vi "Build Test Sequence.vi"(8 "error in":errorcluster, 11 "Configured Steps In":T1[](array[typedef])) -> (0 "error out":errorcluster, 3 "Configured Steps Out":T1[](array[typedef]))   [LabVIEW 2018]
doc: "This VI provides a UI to build, configure, and modify a real-time control sequence."
uses:
  controls/Configured Step.ctl
  controls/VI Reference Type.ctl
panel:
  in  "Save":bool
  in  "Load":bool
  in  "Cancel Button":bool
  in  "Move Down":bool
  in  "Move Up":bool
  in  "Done":bool
  in  "Add Step":bool
  in  "Remove Step":bool
  in  "Control Sequence":i32(listbox)
  in  "Available Steps":i32(listbox)
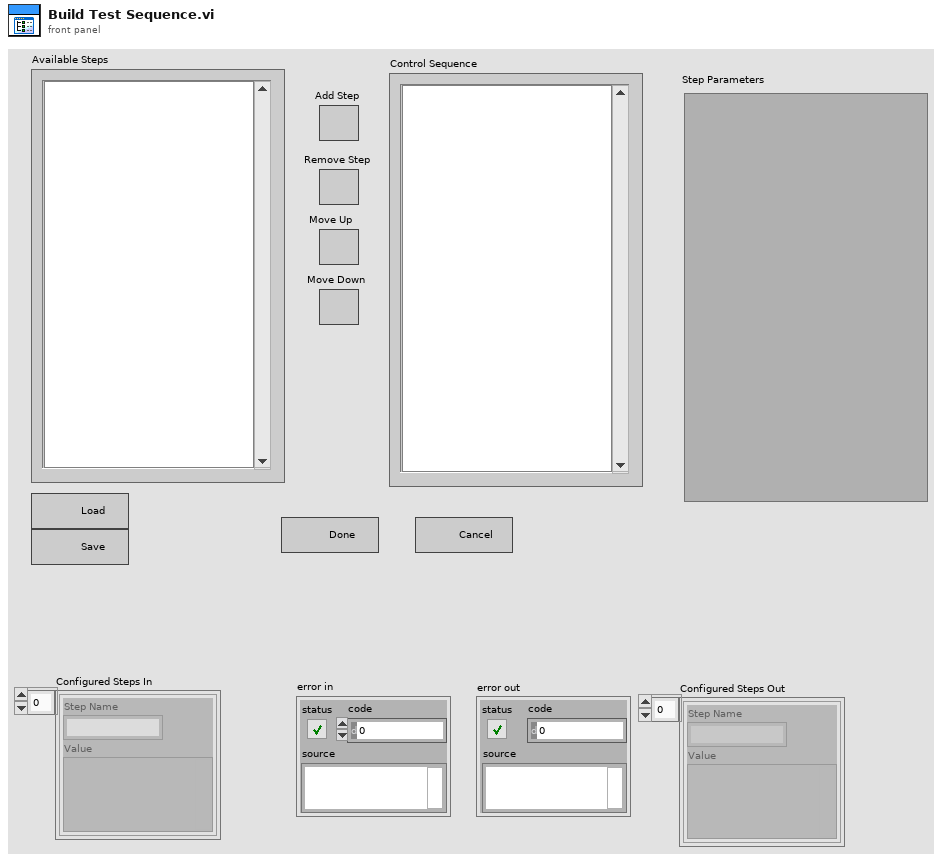
[diagram p1: front panel]
types:
  T1 = typedef "Configured Step.ctl" = cluster{"Step Name":string, "Value":variant}
  T2 = typedef "VI Reference Type.ctl" = refnum<vi>
  T3 = enum16{"open", "replace", "create", "open or create", "replace or create", "replace or create with confirmation"}
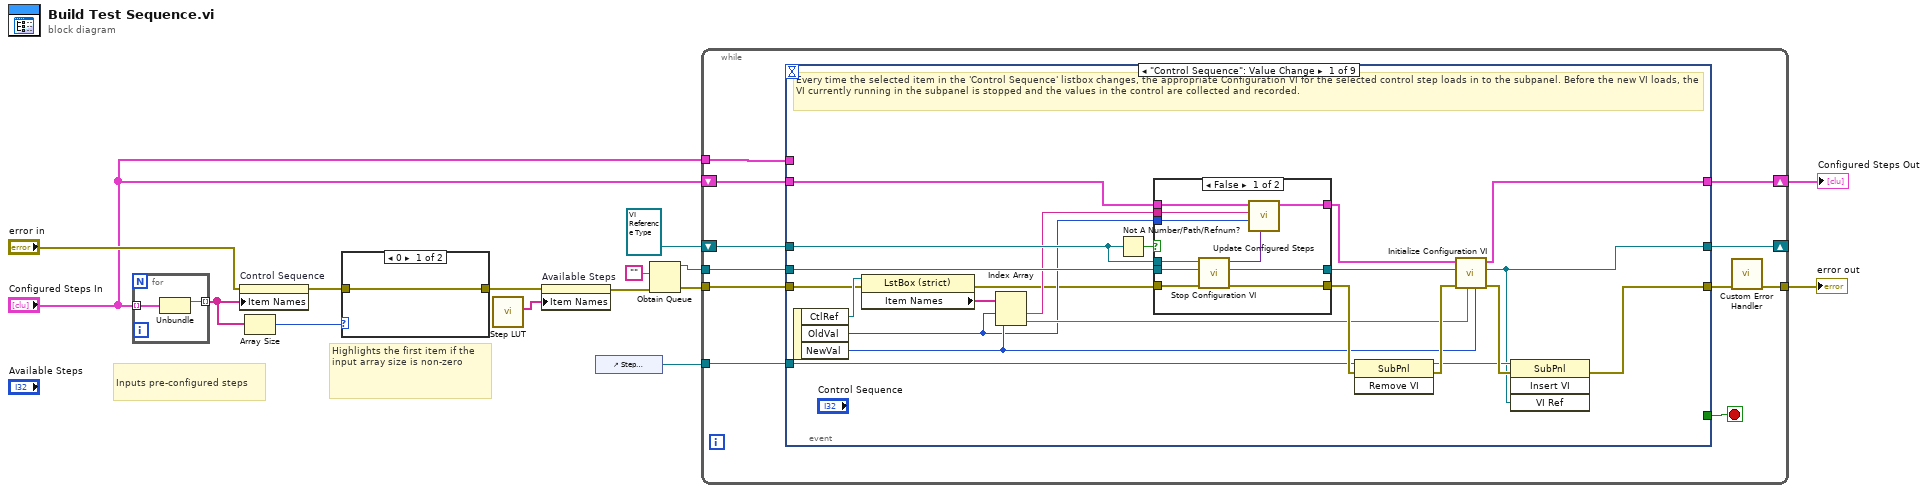
[diagram p0: block diagram]
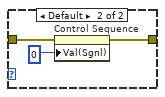
[diagram p2: hidden frame]
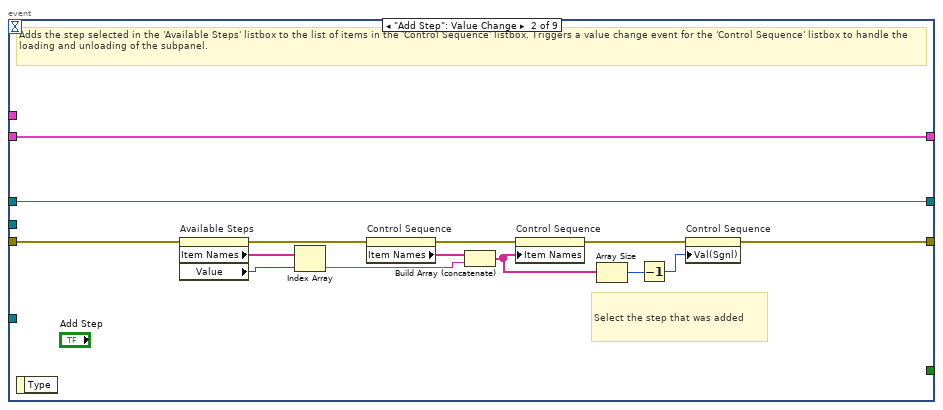
[diagram p4: hidden frame]
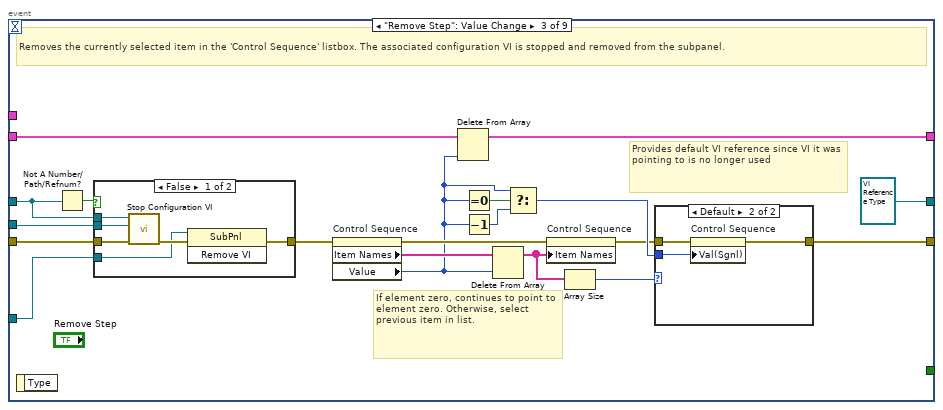
[diagram p5: hidden frame]
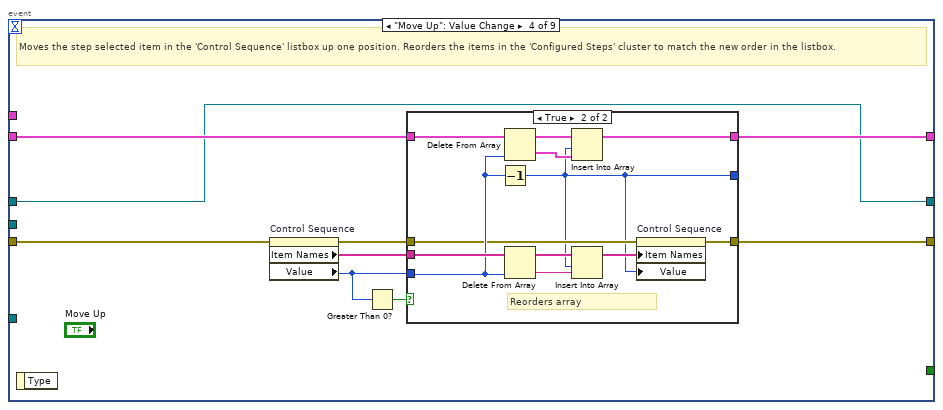
[diagram p8: hidden frame]
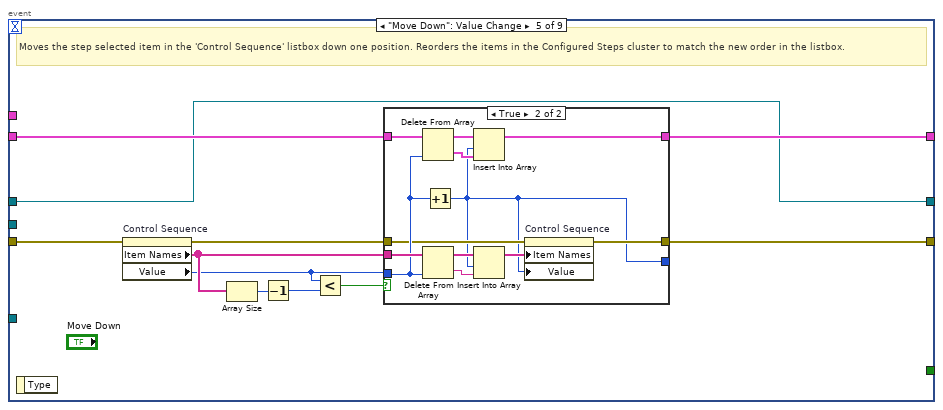
[diagram p10: hidden frame]
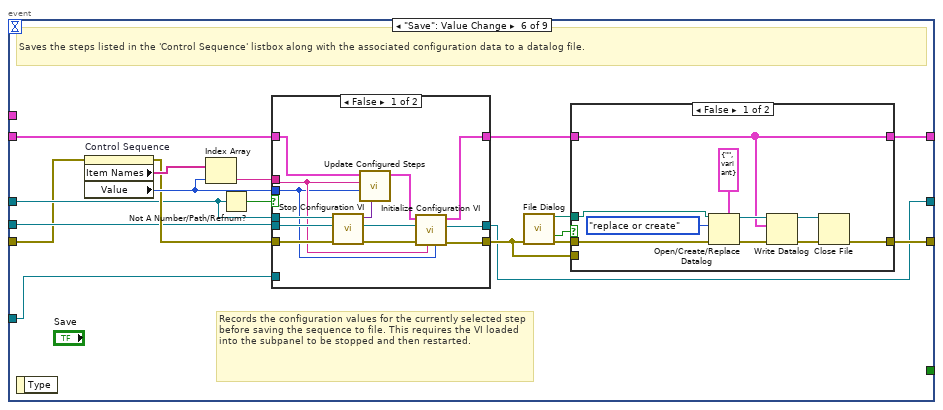
[diagram p12: hidden frame]
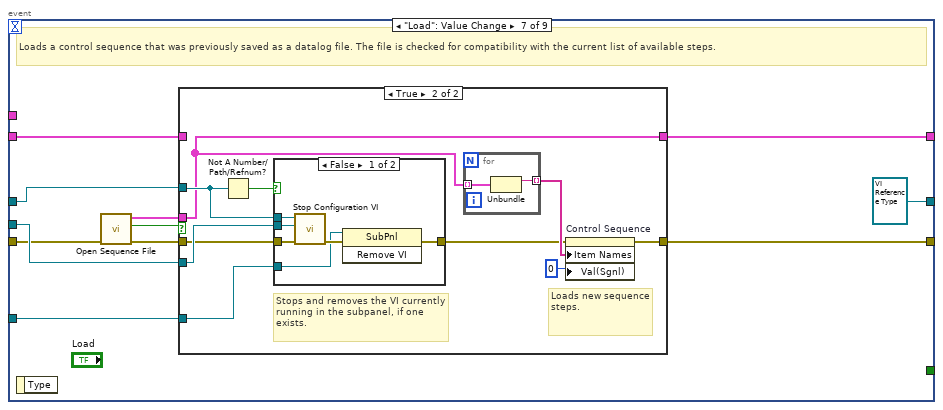
[diagram p15: hidden frame]
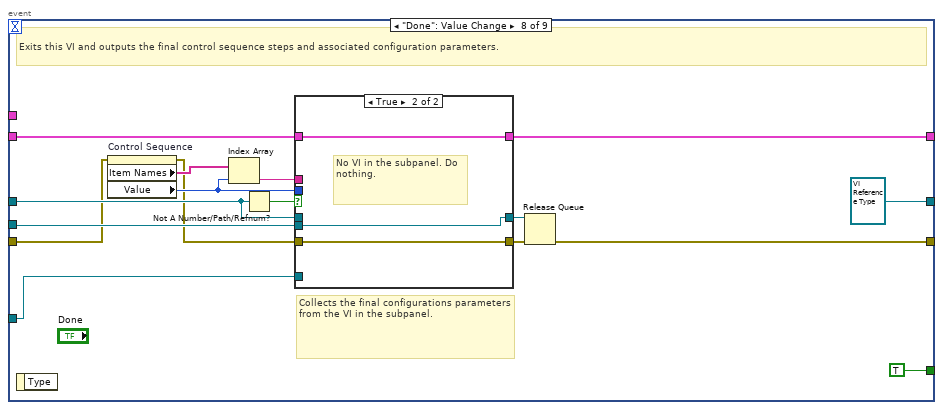
[diagram p18: hidden frame]
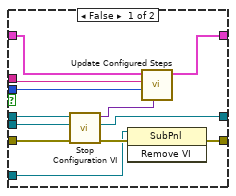
[diagram p19: hidden frame]
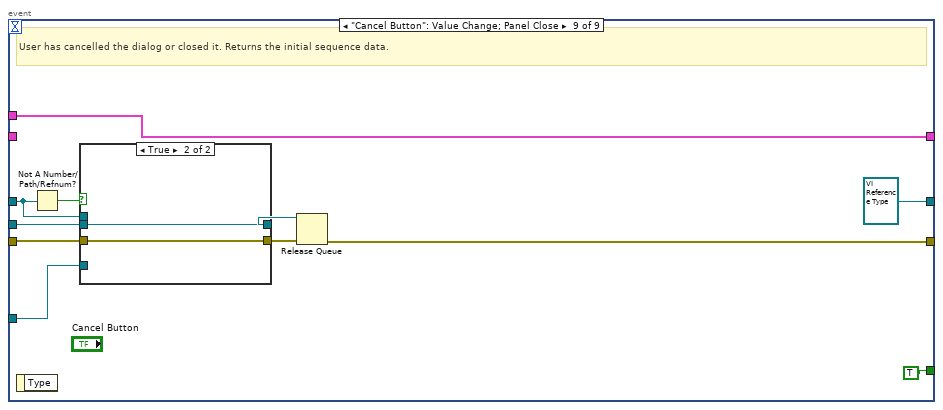
[diagram p20: hidden frame]
diagram:
  # "Highlights the first item if the input array size is non-zero"
  # "Inputs pre-configured steps"
  n1 = for {
    tunnel: "Configured Steps In" -> [w17] mode=indexing
    tunnel: [w16] -> w13 mode=indexing
    n2 = Unbundle(w17) -> ("Step Name"=w16:string)  [unwired: 1 out]
  }
  n3 = property on="Control Sequence" class="LstBox (strict)"(error in="error in", "Item Names"=w13) -> (error out=w10:errorcluster)  [unwired: 1 in, 1 out]
  n4 = Array Size(array=w13) -> (size(s)=w1:i32)
  n5 = case shown="0" w1 {
    tunnel: w10 -> [w18 w20]
    tunnel: [w18 w19] -> w9
    frame 0 {
    }
    frame Default {
      n6 = property on="Control Sequence" class="LstBox (strict)"(error in=w20, "Val(Sgnl)"=0 ("Value (Signaling)")) -> (error out=w19:errorcluster)  [unwired: 1 in, 1 out]
    }
  }
  n7 = call "Step LUT.vi"() -> ("Available Steps"=w8:string[])  [unwired: 10 in, 1 out]
  n8 = property on="Available Steps" class="LstBox (strict)"(error in=w9, "Item Names"=w8) -> (error out=w7:errorcluster)  [unwired: 1 in, 1 out]
  n9 = control-ref of="Step Parameters"() -> (w14:refnum<vi>)
  n10 = Obtain Queue(element data type="", error in (no error)=w7) -> (queue out=w4:refnum<queue>, error out=w6:errorcluster)  [unwired: 3 in, 1 out]
  n11 = while {
    shift-right: [w25] -> _
    shift-left: T2 refnum ("VI reference") -> [w31]
    shift-right: [w30] -> w12
    shift-left: "Configured Steps In" -> [w29]
    tunnel: w14 -> [w22]
    tunnel: "Configured Steps In" -> [w27]
    tunnel: w4 -> [w26]
    tunnel: w6 -> [w28]
    tunnel: [w23] -> w15
    stop <- w32 stop-if-true
    n12 = event shown="[0] \"Control Sequence\": Value Change" {
      selector: _ -> [_ _ _ _ _ _ _ _ _]
      dyn-events: _ -> [_ _ _ _ _ _ _ _ _]
      timeout: _ -> [_ _ _ _ _ _ _ _ _]
      tunnel: [_ _ _ _ _ _ _ TRUE TRUE] -> w32
      tunnel: w31 -> [w51 w70 w91 w112 w139 w165 w213 w250 w276]
      tunnel: [w41 w79 w98 w117 w144 w175 w218 w248 w281] -> w30
      tunnel: w29 -> [w50 w79 w97 w118 w145 w168 w212 w247 _]
      tunnel: w28 -> [w39 w71 w89 w120 w146 w164 w211 w241 w275]
      tunnel: [w44 w75 w82 w115 w142 w179 w217 w254 w279] -> w24
      tunnel: w22 -> [w48 _ w88 _ _ w169 w216 w245 w274]
      tunnel: w27 -> [_ _ _ _ _ _ _ _ w281]
      tunnel: w26 -> [w43 _ w90 _ _ w166 w214 w251 w272]
      tunnel: [w40 w70 T2 refnum ("VI Reference out") w112 w139 w162 T2 refnum ("VI reference in") T2 refnum ("VI reference in") T2 refnum ("VI reference in")] -> w25
      event "Control Sequence": Value Change {
        # "Every time the selected item in the 'Control Sequence' listbox changes, the appropriate Configuration VI for the selected control step loads in to the subpanel. Before the new VI loads, the VI currently running in the subpanel is stopped and the values in the control are collected and recorded."
        n13 = event-data() -> ("CtlRef"=w54:refnum<vi>, "OldVal"=w35:i32, "NewVal"=w37:i32)  [unwired: 1 in]
        n14 = property class="LstBox (strict)"(reference=w54, error in=w39) -> (error out=w33:errorcluster, "Item Names"=w53:string[])  [unwired: 1 out]
        n15 = Index Array(array=w53, index #1=w35, index #2=w37) -> (element #1=w36:string, element #2=w38:string)
        n16 = Not A Number/Path/Refnum?(number/path/refnum=w51) -> (NaN/Path/Refnum?=w52:bool)
        n17 = case shown="False" w52 {
          tunnel: w51 -> [w64 _]
          tunnel: w36 -> [w59 _]
          tunnel: w50 -> [w56 w65]
          tunnel: [w62 w67] -> w49
          tunnel: w35 -> [w60 _]
          tunnel: w33 -> [w63 w67]
          tunnel: w43 -> [w61 w66]
          tunnel: [w58 w66] -> w42
          tunnel: [w55 w65] -> w34
          frame False {
            n18 = call "Stop Configuration VI.vi"("error in (no error)"=w63, "Subpanel Queue In"=w61, "VI in"=w64) -> ("error out"=w62:errorcluster, "Subpanel Queue Out"=w58:refnum<queue>, "Variant Out"=w57:variant)  [unwired: 6 in]
            n19 = call "Update Configured Steps.vi"("Parameters In"=w57, "Step Number"=w60, "Step Name"=w59, "Configured Steps In"=w56) -> ("Configured Steps Out"=w55:T1[])  [unwired: 7 in]
          }
          frame True {
            # "No VI currently loaded in the subpanel. Do nothing"
          }
        }
        n20 = invoke class="SubPnl" method="Remove VI"(reference=w48, error in=w49) -> (reference out=w45:refnum<vi>, error out=w47:errorcluster)  [unwired: 1 in, 1 out]
        n21 = call "Initialize Configuration VI.vi"("Step Number"=w37, "Step Name"=w38, "error in (no error)"=w47, "Subpanel Queue in"=w42, "Configured Steps In"=w34) -> ("error out"=w46:errorcluster, "VI Reference out"=w40:T2, "Configured Steps Out"=w41:T1[])  [unwired: 4 in]
        n22 = invoke on="Invoke Node" class="SubPnl" method="Insert VI"(reference=w45, error in=w46, "VI Ref"=w40) -> (error out=w44:errorcluster)  [unwired: 1 in, 3 out]
      }
      event "Add Step": Value Change {
        # "Select the step that was added"
        # "Adds the step selected in the 'Available Steps' listbox to the list of items in the 'Control Sequence' listbox. Triggers a value change event for the 'Control Sequence' listbox to handle the loading and unloading of the subpanel."
        n23 = event-data() -> ()  [unwired: 1 in, 1 out]
        n24 = property on="Available Steps" class="LstBox (strict)"(error in=w71) -> (error out=w78:errorcluster, "Item Names"=w72:string[], "Value"=w69:i32)  [unwired: 1 in, 1 out]
        n25 = Index Array(array=w72, index=w69) -> (element=w73:string)
        n26 = property on="Control Sequence" class="LstBox (strict)"(error in=w78) -> (error out=w77:errorcluster, "Item Names"=w81:string[])  [unwired: 1 in, 1 out]
        n27 = Build Array (concatenate)(w81, w73) -> (w68:string[])
        n28 = property on="Control Sequence" class="LstBox (strict)"(error in=w77, "Item Names"=w68) -> (error out=w76:errorcluster)  [unwired: 1 in, 1 out]
        n29 = Array Size(array=w68) -> (size(s)=w80:i32)
        n30 = Decrement(x=w80) -> (x-1=w74:i32)
        n31 = property on="Control Sequence" class="LstBox (strict)"(error in=w76, "Val(Sgnl)"=w74) -> (error out=w75:errorcluster)  [unwired: 1 in, 1 out]
      }
      event "Remove Step": Value Change {
        # "If element zero, continues to point to element zero. Otherwise, select previous item in list."
        # "Provides default VI reference since VI it was pointing to is no longer used"
        # "Removes the currently selected item in the 'Control Sequence' listbox. The associated configuration VI is stopped and removed from the subpanel."
        n32 = event-data() -> ()  [unwired: 1 in, 1 out]
        n33 = Not A Number/Path/Refnum?(number/path/refnum=w91) -> (NaN/Path/Refnum?=w92:bool)
        n34 = case shown="False" w92 {
          tunnel: w89 -> [w107 w111]
          tunnel: [w110 w111] -> w87
          tunnel: w91 -> [w109 _]
          tunnel: w90 -> [w108 _]
          tunnel: w88 -> [w105 _]
          frame False {
            n35 = call "Stop Configuration VI.vi"("error in (no error)"=w107, "Subpanel Queue In"=w108, "VI in"=w109) -> ("error out"=w106:errorcluster)  [unwired: 6 in, 2 out]
            n36 = invoke class="SubPnl" method="Remove VI"(reference=w105, error in=w106) -> (error out=w110:errorcluster)  [unwired: 1 in, 2 out]
          }
          frame True {
          }
        }
        n37 = property on="Control Sequence" class="LstBox (strict)"(error in=w87) -> (error out=w99:errorcluster, "Item Names"=w100:string[], "Value"=w95:i32)  [unwired: 1 in, 1 out]
        n38 = Delete From Array(array=w97, index=w95) -> (array with subset deleted=w98:T1[])  [unwired: 1 in, 1 out]
        n39 = Equal To 0?(x=w95) -> (x = 0?=w96:bool)
        n40 = Decrement(x=w95) -> (x-1=w94:i32)
        n41 = Delete From Array(array=w100, index=w95) -> (array with subset deleted=w86:string[])  [unwired: 1 in, 1 out]
        n42 = Select(t=w95, s=w96, f=w94) -> (s? t:f=w84:i32)
        n43 = property on="Control Sequence" class="LstBox (strict)"(error in=w99, "Item Names"=w86) -> (error out=w83:errorcluster)  [unwired: 1 in, 1 out]
        n44 = Array Size(array=w86) -> (size(s)=w85:i32)
        n45 = case shown="Default" w85 {
          tunnel: w84 -> [_ w104]
          tunnel: w83 -> [w101 w103]
          tunnel: [w101 w102] -> w82
          frame 0 {
            # "No elements in Control Sequence listbox. Do nothing."
          }
          frame Default {
            n46 = property on="Control Sequence" class="LstBox (strict)"(error in=w103, "Val(Sgnl)"=w104) -> (error out=w102:errorcluster)  [unwired: 1 in, 1 out]
          }
        }
      }
      event "Move Up": Value Change {
        # "Moves the step selected item in the 'Control Sequence' listbox up one position. Reorders the items in the 'Configured Steps' cluster to match the new order in the listbox."
        n47 = event-data() -> ()  [unwired: 1 in, 1 out]
        n48 = property on="Control Sequence" class="LstBox (strict)"(error in=w120) -> (error out=w116:errorcluster, "Item Names"=w119:string[], "Value"=w113:i32)  [unwired: 1 in, 1 out]
        n49 = Greater Than 0?(x=w113) -> (x > 0?=w114:bool)
        n50 = case shown="True" w114 {
          tunnel: w119 -> [_ w135]
          tunnel: w118 -> [w121 w134]
          tunnel: w113 -> [w122 w131]
          tunnel: [w121 w128] -> w117
          tunnel: w116 -> [w123 w127]
          tunnel: [w123 w125] -> w115
          tunnel: [w122 w124] -> _
          frame False {
            # "Selected item is already at the top of the list. Do nothing."
          }
          frame True {
            # "Reorders array"
            n51 = Decrement(x=w131) -> (x-1=w124:i32)
            n52 = Delete From Array(array=w134, index=w131) -> (deleted portion=w129:T1, array with subset deleted=w130:T1[])  [unwired: 1 in]
            n53 = Delete From Array(array=w135, index=w131) -> (deleted portion=w132:string, array with subset deleted=w133:string[])  [unwired: 1 in]
            n54 = Insert Into Array(array=w130, index=w124, new element=w129) -> (w128:T1[])
            n55 = Insert Into Array(array=w133, index=w124, new element=w132) -> (w126:string[])
            n56 = property on="Control Sequence" class="LstBox (strict)"(error in=w127, "Item Names"=w126, "Value"=w124) -> (error out=w125:errorcluster)  [unwired: 1 in, 1 out]
          }
        }
      }
      event "Move Down": Value Change {
        # "Moves the step selected item in the 'Control Sequence' listbox down one position. Reorders the items in the Configured Steps cluster to match the new order in the listbox."
        n57 = event-data() -> ()  [unwired: 1 in, 1 out]
        n58 = property on="Control Sequence" class="LstBox (strict)"(error in=w146) -> (error out=w143:errorcluster, "Item Names"=w140:string[], "Value"=w138:i32)  [unwired: 1 in, 1 out]
        n59 = Array Size(array=w140) -> (size(s)=w141:i32)
        n60 = Decrement(x=w141) -> (x-1=w137:i32)
        n61 = Less?(x=w138, y=w137) -> (x < y?=w136:bool)
        n62 = case shown="True" w136 {
          tunnel: w140 -> [_ w161]
          tunnel: w145 -> [w147 w160]
          tunnel: w138 -> [w148 w157]
          tunnel: [w147 w154] -> w144
          tunnel: w143 -> [w149 w153]
          tunnel: [w149 w151] -> w142
          tunnel: [w148 w150] -> _
          frame False {
            # "Selected item is already the last item in the list. Do nothing."
          }
          frame True {
            n63 = Delete From Array(array=w160, index=w157) -> (deleted portion=w155:T1, array with subset deleted=w156:T1[])  [unwired: 1 in]
            n64 = Delete From Array(array=w161, index=w157) -> (deleted portion=w158:string, array with subset deleted=w159:string[])  [unwired: 1 in]
            n65 = Increment(x=w157) -> (x+1=w150:i32)
            n66 = Insert Into Array(array=w156, index=w150, new element=w155) -> (w154:T1[])
            n67 = Insert Into Array(array=w159, index=w150, new element=w158) -> (w152:string[])
            n68 = property on="Control Sequence" class="LstBox (strict)"(error in=w153, "Item Names"=w152, "Value"=w150) -> (error out=w151:errorcluster)  [unwired: 1 in, 1 out]
          }
        }
      }
      event "Save": Value Change {
        # "Records the configuration values for the currently selected step before saving the sequence to file. This requires the VI loaded into the subpanel to be stopped and then restarted."
        # "Saves the steps listed in the 'Control Sequence' listbox along with the associated configuration data to a datalog file."
        n69 = event-data() -> ()  [unwired: 1 in, 1 out]
        n70 = property on="Control Sequence" class="LstBox (strict)"(error in=w164) -> (error out=w170:errorcluster, "Item Names"=w173:string[], "Value"=w172:i32)  [unwired: 1 in, 1 out]
        n71 = Index Array(array=w173, index=w172) -> (element=w171:string)
        n72 = Not A Number/Path/Refnum?(number/path/refnum=w165) -> (NaN/Path/Refnum?=w174:bool)
        n73 = case shown="False" w174 {
          tunnel: w165 -> [w192 w193]
          tunnel: w171 -> [w184 _]
          tunnel: [w181 w195] -> w167
          tunnel: w168 -> [w188 w195]
          tunnel: [w182 w194] -> w163
          tunnel: w172 -> [w183 _]
          tunnel: w170 -> [w191 w194]
          tunnel: w166 -> [w190 _]
          tunnel: w169 -> [_ _]
          tunnel: [w180 w193] -> w162
          frame False {
            n74 = call "Stop Configuration VI.vi"("error in (no error)"=w191, "Subpanel Queue In"=w190, "VI in"=w192) -> ("error out"=w186:errorcluster, "Subpanel Queue Out"=w187:refnum<queue>, "Variant Out"=w189:variant)  [unwired: 6 in]
            n75 = call "Update Configured Steps.vi"("Parameters In"=w189, "Step Number"=w183, "Step Name"=w184, "Configured Steps In"=w188) -> ("Configured Steps Out"=w185:T1[])  [unwired: 7 in]
            n76 = call "Initialize Configuration VI.vi"("Step Number"=w183, "Step Name"=w184, "error in (no error)"=w186, "Subpanel Queue in"=w187, "Configured Steps In"=w185) -> ("error out"=w182:errorcluster, "VI Reference out"=w180:T2, "Configured Steps Out"=w181:T1[])  [unwired: 4 in]
          }
          frame True {
            # "Not a valid VI reference\n as an input. \nDo nothing"
          }
        }
        n77 = call "File Dialog"("error in"=w163) -> ("selected path"=w177:path, "cancelled"=w176:bool, "error out"=w178:errorcluster)  [unwired: 11 in, 1 out]
        n78 = case shown="False" w176 {
          tunnel: w167 -> [w196 w207]
          tunnel: [w199 w206] -> w179
          tunnel: w178 -> [w198 _]
          tunnel: w177 -> [w197 _]
          tunnel: [w196 w207] -> w175
          tunnel: w163 -> [_ w206]
          frame False {
            n79 = Open/Create/Replace Datalog(5:T1 {"Step Name"="", "Value"=variant} ("Configured Step"), 8:w198, 10:T3."replace or create" ("operation (0:open)"), 11:w197) -> (0:w205:errorcluster, 3:w202:refnum<k1>)  [unwired: 2 in, 1 out]
            n80 = Write Datalog(4:w205, 6:w196, 7:w202) -> (0:w201:errorcluster, 3:w200:refnum<k1>)
            n81 = Close File(refnum=w200, error in=w201) -> (error out=w199:errorcluster)  [unwired: 1 out]
          }
          frame True {
          }
        }
      }
      event "Load": Value Change {
        # "Loads a control sequence that was previously saved as a datalog file. The file is checked for compatibility with the current list of available steps."
        n82 = event-data() -> ()  [unwired: 1 in, 1 out]
        n83 = call "Open Sequence File.vi"("error in"=w211) -> ("error out"=w210:errorcluster, "Valid?"=w209:bool, "Configured Steps Out"=w208:T1[])  [unwired: 8 in]
        n84 = case shown="True" w209 {
          tunnel: [w220 w222] -> w218
          tunnel: [w219 w229] -> w217
          tunnel: w210 -> [w219 w221]
          tunnel: w212 -> [w220 _]
          tunnel: w216 -> [_ w223]
          tunnel: w214 -> [_ w228]
          tunnel: w213 -> [_ w227]
          tunnel: w208 -> [_ w222]
          frame False {
            # "Load cancelled or an invalid datalog file was selected. Do nothing and keep current sequence."
          }
          frame True {
            # "Loads new sequence steps."
            # "Stops and removes the VI currently running in the subpanel, if one exists."
            n85 = Not A Number/Path/Refnum?(number/path/refnum=w227) -> (NaN/Path/Refnum?=w226:bool)
            n86 = case shown="False" w226 {
              tunnel: [w236 w237] -> w225
              tunnel: w227 -> [w235 _]
              tunnel: w228 -> [w233 _]
              tunnel: w221 -> [w232 w237]
              tunnel: w223 -> [w231 _]
              frame False {
                n87 = call "Stop Configuration VI.vi"("error in (no error)"=w232, "Subpanel Queue In"=w233, "VI in"=w235) -> ("error out"=w234:errorcluster)  [unwired: 6 in, 2 out]
                n88 = invoke class="SubPnl" method="Remove VI"(reference=w231, error in=w234) -> (error out=w236:errorcluster)  [unwired: 1 in, 2 out]
              }
              frame True {
              }
            }
            n89 = for {
              tunnel: w222 -> [w239] mode=indexing
              tunnel: [w238] -> w230 mode=indexing
              n90 = Unbundle(w239) -> ("Step Name"=w238:string)  [unwired: 1 out]
            }
            n91 = property on="Control Sequence" class="LstBox (strict)"(error in=w225, "Item Names"=w230, "Val(Sgnl)"=0 ("Value (Signaling)")) -> (error out=w229:errorcluster)  [unwired: 1 in, 1 out]
          }
        }
      }
      event "Done": Value Change {
        # "Collects the final configurations parameters from the VI in the subpanel."
        # "Exits this VI and outputs the final control sequence steps and associated configuration parameters."
        n92 = event-data() -> ()  [unwired: 1 in, 1 out]
        n93 = property on="Control Sequence" class="LstBox (strict)"(error in=w241) -> (error out=w240:errorcluster, "Item Names"=w244:string[], "Value"=w243:i32)  [unwired: 1 in, 1 out]
        n94 = Index Array(array=w244, index=w243) -> (element=w242:string)
        n95 = Not A Number/Path/Refnum?(number/path/refnum=w250) -> (NaN/Path/Refnum?=w252:bool)
        n96 = case shown="True" w252 {
          tunnel: w250 -> [w267 _]
          tunnel: w242 -> [w263 _]
          tunnel: [w256 w270] -> w248
          tunnel: w247 -> [w257 w270]
          tunnel: [w261 w269] -> w249
          tunnel: w243 -> [w264 _]
          tunnel: w240 -> [w266 w269]
          tunnel: w251 -> [w265 w268]
          tunnel: [w260 w268] -> w246
          tunnel: w245 -> [w259 _]
          frame False {
            n97 = call "Stop Configuration VI.vi"("error in (no error)"=w266, "Subpanel Queue In"=w265, "VI in"=w267) -> ("error out"=w262:errorcluster, "Subpanel Queue Out"=w260:refnum<queue>, "Variant Out"=w258:variant)  [unwired: 6 in]
            n98 = invoke class="SubPnl" method="Remove VI"(reference=w259, error in=w262) -> (error out=w261:errorcluster)  [unwired: 1 in, 2 out]
            n99 = call "Update Configured Steps.vi"("Parameters In"=w258, "Step Number"=w264, "Step Name"=w263, "Configured Steps In"=w257) -> ("Configured Steps Out"=w256:T1[])  [unwired: 7 in]
          }
          frame True {
            # "No VI in the subpanel. Do nothing."
          }
        }
        n100 = Release Queue(queue=w246, error in (no error)=w249) -> (error out=w254:errorcluster)  [unwired: 1 in, 2 out]
      }
      event "Cancel Button": Value Change; Panel Close {
        # "User has cancelled the dialog or closed it. Returns the initial sequence data."
        n101 = event-data() -> ()  [unwired: 1 in, 1 out]
        n102 = Not A Number/Path/Refnum?(number/path/refnum=w276) -> (NaN/Path/Refnum?=w277:bool)
        n103 = case shown="True" w277 {
          tunnel: [w288 w290] -> w273
          tunnel: w276 -> [w287 _]
          tunnel: w272 -> [w285 w289]
          tunnel: w275 -> [w284 w290]
          tunnel: w274 -> [w283 _]
          tunnel: [w282 w289] -> w271
          frame False {
            # "Stops the VI running in the subpanel"
            n104 = call "Stop Configuration VI.vi"("error in (no error)"=w284, "Subpanel Queue In"=w285, "VI in"=w287) -> ("error out"=w286:errorcluster, "Subpanel Queue Out"=w282:refnum<queue>)  [unwired: 6 in, 1 out]
            n105 = invoke class="SubPnl" method="Remove VI"(reference=w283, error in=w286) -> (error out=w288:errorcluster)  [unwired: 1 in, 2 out]
          }
          frame True {
          }
        }
        n106 = Release Queue(queue=w271, error in (no error)=w273) -> (error out=w279:errorcluster)  [unwired: 1 in, 2 out]
      }
    }
    n107 = call "Custom Error Handler.vi"("error in"=w24) -> ("error out"=w23:errorcluster)  [unwired: 10 in]
  }
  "error out" <- w15
  "Configured Steps Out" <- w12
